vi "Read.vi"(8 "error in":errorcluster, 11 "Scanner reference in":refnum<visa-resource-name>) -> (0 "error out":errorcluster, 1 "Scan OK":bool, 2 "Scanned value":string, 3 "Scanner reference out":refnum<visa-resource-name>)   [LabVIEW 2023, in "HoneywellScanner.lvlib"]
uses:
  HoneywellScanner.lvlib
  75488dd3-f4ec-4771-bf02-d410e948b7b7.vi
  28352091-3b78-4962-9b4f-736fd858179a.vi
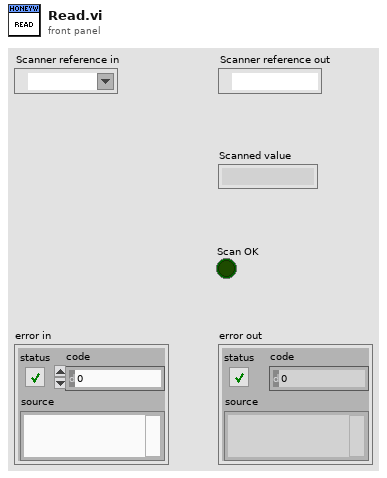
[diagram p1: front panel]
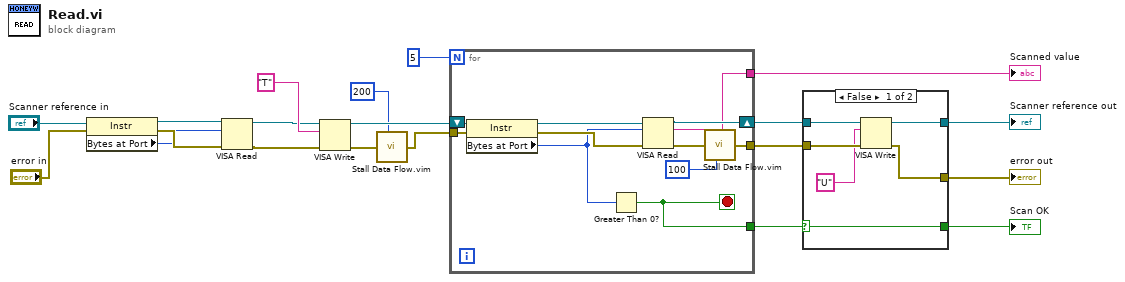
[diagram p0: block diagram]
diagram:
  n1 = property class="Instr"(reference="Scanner reference in", error in="error in") -> (reference out=w7:refnum<visa-resource-name>, error out=w6:errorcluster, "Bytes at Port"=w5:u32)
  n2 = VISA Read(VISA resource name=w7, byte count=w5, error in (no error)=w6) -> (VISA resource name out=w3:refnum<visa-resource-name>, error out=w1:errorcluster)  [unwired: 2 out]
  n3 = VISA Write(VISA resource name=w3, write buffer="T", error in (no error)=w1) -> (VISA resource name out=w19:refnum<visa-resource-name>, error out=w18:errorcluster)  [unwired: 1 out]
  n4 = call "Stall Data Flow.vim"("value in"=w18, "milliseconds to wait"=u32 200) -> ("value out"=w17:errorcluster)  [unwired: 1 out]
  n5 = for {
    N: 5 -> [_]
    tunnel: w17 -> [w28]
    shift-right: [w27] -> w12
    shift-left: w19 -> [w31]
    tunnel: [w22] -> w11
    tunnel: [w24] -> w14
    tunnel: [w23] -> w13
    stop <- w23 stop-if-true
    n6 = property class="Instr"(reference=w31, error in=w28) -> (reference out=w30:refnum<visa-resource-name>, error out=w29:errorcluster, "Bytes at Port"=w26:u32)
    n7 = Greater Than 0?(x=w26) -> (x > 0?=w23:bool)
    n8 = VISA Read(VISA resource name=w30, byte count=w26, error in (no error)=w29) -> (VISA resource name out=w27:refnum<visa-resource-name>, read buffer=w24:string, error out=w25:errorcluster)  [unwired: 1 out]
    n9 = call "Stall Data Flow.vim"("value in"=w25, "milliseconds to wait"=u32 100) -> ("value out"=w22:errorcluster)  [unwired: 1 out]
  }
  "Scanned value" <- w14
  n10 = case shown="False" w13 {
    selector: w13 -> [w37 w38]
    tunnel: w12 -> [w36 w40]
    tunnel: w11 -> [w34 w39]
    tunnel: [w33 w39] -> w10
    tunnel: [w35 w40] -> w9
    tunnel: [w37 w38] -> w8
    frame False {
      n11 = VISA Write(VISA resource name=w36, write buffer="U", error in (no error)=w34) -> (VISA resource name out=w35:refnum<visa-resource-name>, error out=w33:errorcluster)  [unwired: 1 out]
    }
    frame True {
    }
  }
  "Scan OK" <- w8
  "Scanner reference out" <- w9
  "error out" <- w10
